vi "Process.vi"(8 "error in (no error)":errorcluster, 10 "Pound in":refnum<class "Pound.lvclass">, 11 "Qbus in":refnum<class "Qbus.lvclass">) -> (0 "error out":errorcluster)   [LabVIEW 2017, in "McsaAnalysisLowUpdate.lvlib"]
doc: "Calculates features, such as MCSA Speed and Rotor Bar Sideband, from waveforms that the channels in a data group acquire. Subsequent processes can evaluate this feature data to trigger alarms, collect data sets, and perform other operations."
uses:
  <vilib>/addons/InsightCM/Devices/Shared/Mcsa/McsaAnalysisLowUpdate/McsaAnalysisLowUpdate.lvlib
  <vilib>/addons/Qbus/Qbus.lvclass
  <vilib>/NI/Software Watchdog/Pound/Pound.lvclass
  <vilib>/addons/InsightCM/Devices/Shared/Mcsa/McsaAnalysisLowUpdate/controls/Config.ctl
  <vilib>/addons/InsightCM/Devices/Shared/Mcsa/McsaAnalysisLowUpdate/controls/Group.ctl
  <vilib>/addons/InsightCM/Utilities/Analysis/MCSA/controls/McsaLowUpdateChannel.ctl
  <vilib>/addons/InsightCM/Utilities/Analysis/Shared/controls/Feature.ctl
  <vilib>/addons/InsightCM/Utilities/Analysis/Shared/controls/AmplitudeScale.ctl
  <vilib>/addons/InsightCM/Utilities/Analysis/MCSA/controls/McsaMotor.ctl
  <vilib>/addons/InsightCM/Utilities/Analysis/MCSA/controls/McsaCalculationCache.ctl
  <vilib>/addons/Electrical Power/Motor Monitoring/subVIs/ep_Initial Conditions for MCSA Spectra.ctl
  <vilib>/addons/Electrical Power/Motor Monitoring/subVIs/ep_Demodulation Algorithm.ctl
  <vilib>/addons/Electrical Power/Motor Monitoring/subVIs/ep_Zoom FFT Settings.ctl
  <vilib>/addons/Electrical Power/Motor Monitoring/subVIs/ep_Initial Conditions for Speed Estimation.ctl
  <vilib>/NI/Software Watchdog/Watchdog/Watchdog.lvclass
  <vilib>/addons/InsightCM/Devices/Shared/Common/DataFlow/DataFlow.lvlib
  <vilib>/addons/InsightCM/Utilities/GlobalConfiguration/GlobalConfiguration.lvlib
  <vilib>/addons/InsightCM/Utilities/Analysis/Shared/AnalysisHelper.lvlib
  <vilib>/addons/InsightCM/Utilities/Analysis/MCSA/McsaAnalysisFunctions.lvlib
  <vilib>/addons/InsightCM/Devices/Shared/Mcsa/McsaResourceScheduler/McsaResourceScheduler.lvlib
  <vilib>/addons/Electrical Power/Motor Monitoring/NI_EP_Motor Monitoring.lvlib
  <vilib>/addons/TraceLogger/TraceLogger.lvlib
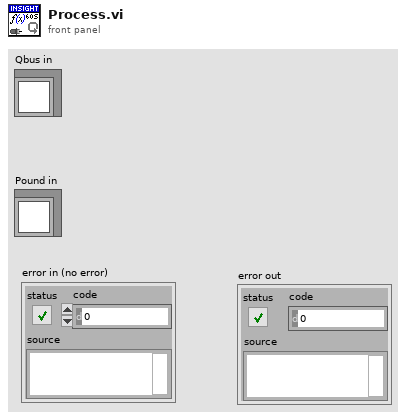
[diagram p1: front panel]
types:
  T1 = typedef "McsaAnalysisLowUpdate.lvlib/Config.ctl" = cluster{"Device Name":string, "Groups":T2[]}
  T2 = typedef "McsaAnalysisLowUpdate.lvlib/Group.ctl" = cluster{"Name":string, "Channels":T3[], "Motor Information":T6, "Calculation Cache":T7}
  T3 = typedef "McsaAnalysisFunctions.lvlib/McsaLowUpdateChannel.ctl" = cluster{"Name":string, "Id":string, "Type":string, "Wiring Configuration":string, "Nominal Voltage":dbl, "Phase A Channel":string, "Phase B Channel":string, "Phase C Channel":string, "Channel Status":string, "Features":T4[], "Data Valid":bool, "Acq Timestamp":timestamp}
  T4 = typedef "AnalysisHelper.lvlib/Feature.ctl" = cluster{"MetricType":string, "TdmsPropName":string, "DisplayName":string, "Unit":string, "Use Volts":bool, "Value":dbl, "Tag Id":string, "Properties":variant, "Amplitude Scale":T5, "valid":bool}
  T5 = typedef "AnalysisHelper.lvlib/AmplitudeScale.ctl" = enum16{"rms", "peak", "pk-pk"}
  T6 = typedef "McsaAnalysisFunctions.lvlib/McsaMotor.ctl" = cluster{"Model":string, "Manufacturer":string, "Serial Number":string, "Horsepower":dbl, "Horsepower Unit":string, "Full Load Speed":dbl, "Synchronous Speed":dbl, "Rated Volts":dbl, "Full Load Amps":dbl, "Frequency":dbl, "Service Factor":dbl, "Efficiency":dbl, "Efficiency @ 75% Load":dbl, "Efficiency @ 50% Load":dbl, "Efficiency @ 25% Load":dbl, "Power Factor":dbl, "VoltageBus":string, "VoltageBus ID":string, "Stator Resistance":dbl, "Estimate Stator Resistance":bool}
  T7 = typedef "McsaAnalysisFunctions.lvlib/McsaCalculationCache.ctl" = cluster{"Spectrum Reset":bool, "Spectrum":cluster{"f0":dbl, "df":dbl, "magnitude [dB]":dbl[]}, "max sideband magnitude [dB]":dbl, "rotor sideband step [Hz]":dbl, "spectrum initial conditions":T8, "Speed Reset":bool, "speed [RPM]":dbl, "slip":dbl, "speed initial conditions":T11, "line frequency [Hz]":dbl}
  T8 = typedef "NI_EP_Motor Monitoring.lvlib/ep_Initial Conditions for MCSA Spectra.ctl" = cluster{"hilbert state":cluster{"delay conditions":dbl[], "filter conditions":dbl[]}, "zoom FFT state":cluster{"phase state":dbl, "zoom FFT state":cluster{"zoom settings state":cluster{"zoom":i32, "stop band attenuation":enum16{"84 dB", "96 dB", "120 dB"}, "alias protect in final transition":bool, "oversampling ratio":dbl}, "SML Decimation Filter (complex input) state":cluster{"decimation settings state":cluster{"M":i32, "stop band attenuation":enum16{"84 dB", "96 dB", "120 dB"}, "alias protect in transition band":bool, "oversampling ratio":dbl}, "counter for garbage samples state":i32, "sml_Parameter Setting for Zoom Factor state":cluster{"filter length * interpolation state":i32, "interpolation state":i32, "comb filter order state":i32, "CFIR par state":cluster{"h":dbl[], "M":i32, "N":i32}, "LFIR par state":cluster{"h":dbl[], "M":i32, "N":i32}, "CIC Stages state":i32}, "aal_CIC (complex input) state":cluster{"aal_cascaded moving average (complex input) state":cluster{"states":cdb[], "circular buffers state":cdb[][], "circular buffer counter state":i32}, "aal_moving average with decimation by order (complex input) state":cluster{"residue result state":cdb, "processed data counter state":i32}}, "sml_Cascaded Decimation Filter (complex input) CFIR state":cluster{"unprocessed data state":cdb[], "final conditions state":cdb[][], "sml_M-1 Decimator with IC (complex input) state":cluster{"coefficients in reverse order state":dbl[], "max index for coefficients state":i32}}, "sml_Cascaded Decimation Filter (complex input) LFIR state":cluster{"unprocessed data state":cdb[], "final conditions state":cdb[][], "sml_M-1 Decimator with IC (complex input) state":cluster{"coefficients in reverse order state":dbl[], "max index for coefficients state":i32}}}, "ma_SML Data Packing (complex input) state":cluster{"array getting packed state":cdb[], "last array processed state":cdb[], "index state":i32, "packing parameters state":cluster{i32, "size":i32}}}, "FFT{X} [Vrms]":cdb[]}, "IIR filter state":cluster{"filter state":dbl[]}, "demodulation settings":cluster{"enable? (F)":bool, "algorithm":T9}, "highpass IIR Filter":cluster{"filter structure":enum32{"IIR 2nd Order", "IIR 4th Order"}, "Reverse Coefficients":dbl[], "Forward Coefficients":dbl[]}, "Hilbert FIR filter":cluster{"coefficients":dbl[], "delay":i32}, "zoom FFT settings":T10}
  T9 = typedef "NI_EP_Motor Monitoring.lvlib/ep_Demodulation Algorithm.ctl" = enum16{"1-phase signal", "3-phase signals"}
  T10 = typedef "NI_EP_Motor Monitoring.lvlib/ep_Zoom FFT Settings.ctl" = cluster{"FFT settings":cluster{"window":u16, "Window Size":i32, "FFT Size":i32, "%overlap":dbl}, "zoom settings":cluster{"zoom":i32, "stop band attenuation":enum16{"84 dB", "96 dB", "120 dB"}, "alias protect in final transition":bool, "oversampling ratio":dbl}, "other settings":cluster{"fmod":dbl, "f0":dbl, "df":dbl, "oidx":i32, "olen":i32}, "iterations":i32, "max block size":i32, "fs":dbl}
  T11 = typedef "NI_EP_Motor Monitoring.lvlib/ep_Initial Conditions for Speed Estimation.ctl" = cluster{"SVAF state":cluster{"space vector amplitude":dbl, "hilbert state":cluster{"delay conditions":dbl[], "filter conditions":dbl[]}}, "zoom FFT state":cluster{"phase state":dbl, "zoom FFT state":cluster{"zoom settings state":cluster{"zoom":i32, "stop band attenuation":enum16{"84 dB", "96 dB", "120 dB"}, "alias protect in final transition":bool, "oversampling ratio":dbl}, "SML Decimation Filter (complex input) state":cluster{"decimation settings state":cluster{"M":i32, "stop band attenuation":enum16{"84 dB", "96 dB", "120 dB"}, "alias protect in transition band":bool, "oversampling ratio":dbl}, "counter for garbage samples state":i32, "sml_Parameter Setting for Zoom Factor state":cluster{"filter length * interpolation state":i32, "interpolation state":i32, "comb filter order state":i32, "CFIR par state":cluster{"h":dbl[], "M":i32, "N":i32}, "LFIR par state":cluster{"h":dbl[], "M":i32, "N":i32}, "CIC Stages state":i32}, "aal_CIC (complex input) state":cluster{"aal_cascaded moving average (complex input) state":cluster{"states":cdb[], "circular buffers state":cdb[][], "circular buffer counter state":i32}, "aal_moving average with decimation by order (complex input) state":cluster{"residue result state":cdb, "processed data counter state":i32}}, "sml_Cascaded Decimation Filter (complex input) CFIR state":cluster{"unprocessed data state":cdb[], "final conditions state":cdb[][], "sml_M-1 Decimator with IC (complex input) state":cluster{"coefficients in reverse order state":dbl[], "max index for coefficients state":i32}}, "sml_Cascaded Decimation Filter (complex input) LFIR state":cluster{"unprocessed data state":cdb[], "final conditions state":cdb[][], "sml_M-1 Decimator with IC (complex input) state":cluster{"coefficients in reverse order state":dbl[], "max index for coefficients state":i32}}}, "ma_SML Data Packing (complex input) state":cluster{"array getting packed state":cdb[], "last array processed state":cdb[], "index state":i32, "packing parameters state":cluster{i32, "size":i32}}}, "FFT{X} [Vrms]":cdb[]}, "speed state":cluster{"speed [RPM]":dbl, "slip":dbl}, "speed estimation settings":cluster{"% overlap":dbl, "algorithm":T9}, "filter information":cluster{"coefficients":dbl[], "order":i32}, "zoom FFT settings":T10, "last valid window":i32, "fund. frequency for averager":dbl[]}
  T12 = typedef "DataFlow.lvlib/Data.ctl" = cluster{"DataGroup":string, "Waveforms":T13, "Map":T14, "Type":T15}
  T13 = typedef "wfmSGL_DVR.ctl" = refnum<data-value>
  T14 = typedef "PointValueMap.lvlib/PointMap.ctl" = refnum<data-value>
  T15 = typedef "DataFlow.lvlib/Type.ctl" = enum16{"High Rate", "Low Rate", "Burst Mode"}
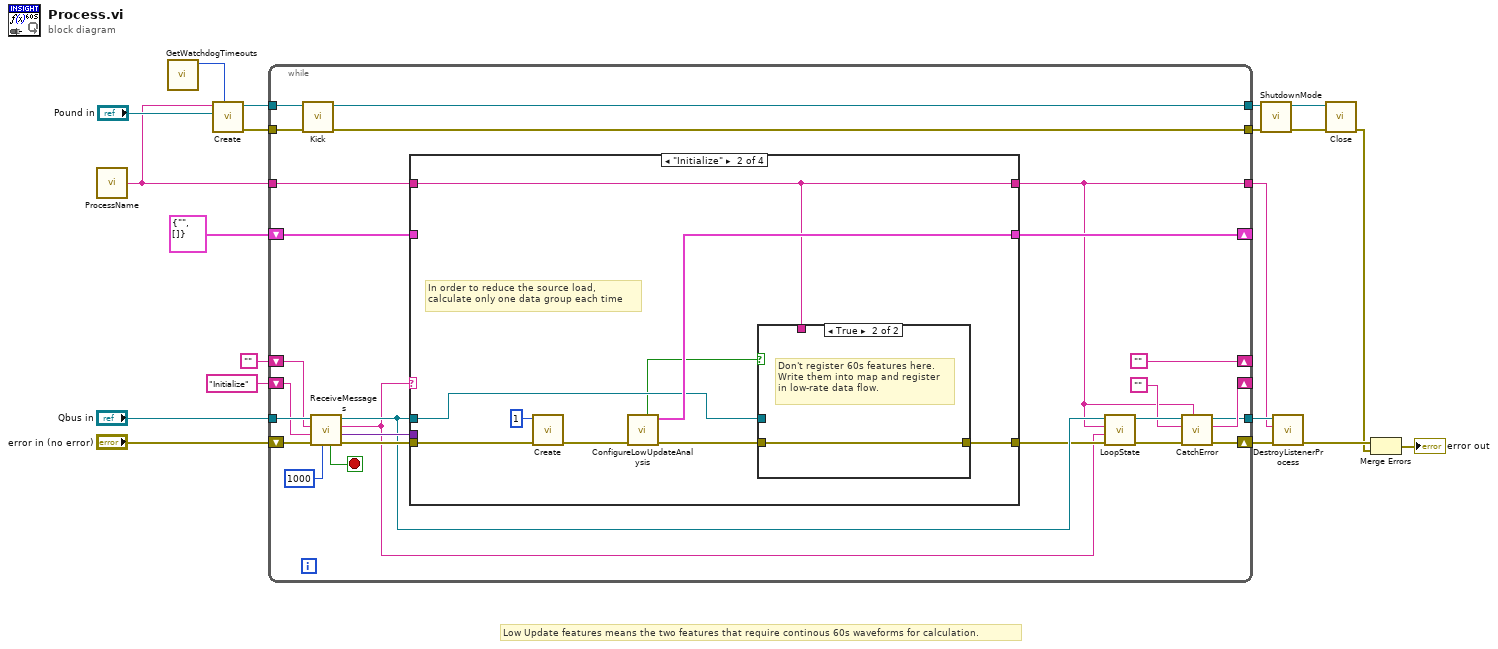
[diagram p0: block diagram]
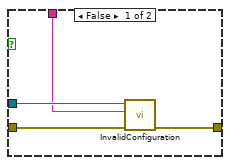
[diagram p3: hidden frame]
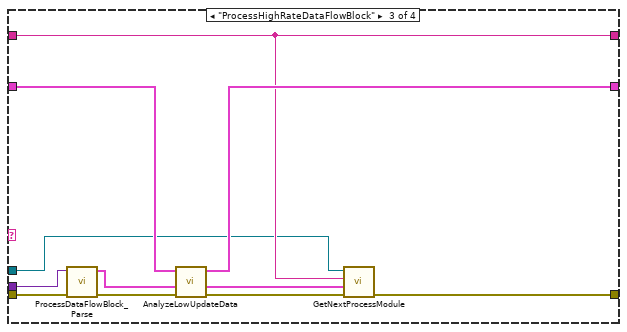
[diagram p4: hidden frame]
diagram:
  # "Low Update features means the two features that require continous 60s waveforms for calculation."
  n1 = call <vilib>:"ProcessName.vi"() -> ("ProcessName"=w2:string)  [unwired: 5 in]
  n2 = call <vilib>:"GetWatchdogTimeouts.vi"() -> ("software timeout"=w3:u32)  [unwired: 10 in, 1 out]
  n3 = call <vilib>:"Create.vi"("Execution Timeout (ms)"=w3, "Pound"="Pound in", "Name"=w2) -> ("error out"=w10:errorcluster, "Watchdog"=w11:refnum<data-value>)  [unwired: 7 in]
  n4 = while {
    shift-right: [""] -> _
    shift-left: "" -> [w40]
    shift-right: [w46] -> _
    shift-left: T1 {"Device Name"="", "Groups"=[]} ("Analysis Configuration") -> [w45]
    shift-right: [w27] -> _
    shift-left: "Initialize" ("MsgName") -> [w38]
    tunnel: w2 -> [w33]
    tunnel: [w26] -> w16
    tunnel: [w24] -> w15
    tunnel: "Qbus in" -> [w43]
    tunnel: [w37] -> w13
    tunnel: [w36] -> w12
    tunnel: w11 -> [w35]
    tunnel: w10 -> [w34]
    shift-right: [w25] -> w17
    shift-left: "error in (no error)" -> [w39]
    stop <- w22 stop-if-true
    n5 = call <vilib>:"Kick.vi"("error in (no error)"=w34, "Watchdog"=w35) -> ("error out"=w37:errorcluster, "Watchdog"=w36:refnum<data-value>)  [unwired: 8 in]
    n6 = call <vilib>:"ReceiveMessages.vi"("Timeout(100)"=1000, "error in (no error)"=w39, "Priority Action"=w38, "Default Action"=w40, "Qbus in"=w43) -> ("error out"=w41:errorcluster, "MsgValue"=w42:variant, "Action"=w23:string, "Qbus out"=w32:refnum<class "Qbus.lvclass">, "Exit"=w22:bool)  [unwired: 2 in]
    n7 = case shown="\"Initialize\"" w23 {
      tunnel: w41 -> [w49 w51 w72 w76]
      tunnel: [w49 w55 w67 w76] -> w31
      tunnel: w42 -> [_ _ w71 _]
      tunnel: [w48 w58 w73 w75] -> w46
      tunnel: w45 -> [w48 _ w74 w75]
      tunnel: w32 -> [_ w57 w66 _]
      tunnel: [w47 w53 w68 w77] -> w24
      tunnel: w33 -> [w47 w53 w68 w77]
      frame Default {
      }
      frame "Initialize" {
        # "In order to reduce the source load, \ncalculate only one data group each time"
        n8 = call <vilib>:"Create.vi"("error in (no error)"=w51, "count"=1) -> ("error out"=w50:errorcluster)  [unwired: 9 in]
        n9 = call <vilib>:"ConfigureLowUpdateAnalysis.vi"("error in (no error)"=w50) -> ("error out"=w56:errorcluster, "analysis config"=w58:T1, "all config found?"=w54:bool)  [unwired: 8 in]
        n10 = case shown="True" w54 {
          tunnel: w57 -> [w62 _]
          tunnel: w56 -> [w61 w63]
          tunnel: [w60 w63] -> w55
          tunnel: w53 -> [w59 _]
          frame False {
            n11 = call <vilib>:"InvalidConfiguration.vi"("error in (no error)"=w61, "description"=w59, "Qbus in"=w62) -> ("error out"=w60:errorcluster)  [unwired: 7 in, 1 out]
          }
          frame True {
            # "Don't register 60s features here.\nWrite them into map and register\nin low-rate data flow."
          }
        }
      }
      frame "ProcessHighRateDataFlowBlock" {
        n12 = call <vilib>:"ProcessDataFlowBlock_Parse.vi"("error in (no error)"=w72, "body"=w71) -> ("error out"=w65:errorcluster, "data"=w69:T12)  [unwired: 8 in]
        n13 = call <vilib>:"AnalyzeLowUpdateData.vi"("error in (no error)"=w65, "data in"=w69, "Analysis Configuration In"=w74) -> ("error out"=w64:errorcluster, "data out"=w70:T12, "Analysis Configuration Out"=w73:T1)  [unwired: 6 in]
        n14 = call <vilib>:"GetNextProcessModule.vi"("error in (no error)"=w64, "data"=w70, "source"=w68, "Qbus in"=w66) -> ("error out"=w67:errorcluster)  [unwired: 6 in, 1 out]
      }
      frame "Exit" {
      }
    }
    n15 = call <vilib>:"LoopState.vi"("error in (no error)"=w31, "loop action"=w23, "process name"=w24, "Qbus in"=w32) -> ("error out"=w28:errorcluster, "Qbus out"=w30:refnum<class "Qbus.lvclass">)  [unwired: 6 in]
    n16 = call <vilib>:"CatchError.vi"("source"=w24, "error in (no error)"=w28, "next action in"="", "Qbus in"=w30) -> ("error out"=w25:errorcluster, "next action out"=w27:string, "Qbus out"=w26:refnum<class "Qbus.lvclass">)  [unwired: 5 in]
  }
  n17 = call <vilib>:"ShutdownMode.vi"("error in (no error)"=w13, "Watchdog"=w12) -> ("error out"=w18:errorcluster, "Watchdog"=w19:refnum<data-value>)  [unwired: 8 in]
  n18 = call <vilib>:"DestroyListenerProcess.vi"("error in (no error)"=w17, "process name"=w15, "Qbus in"=w16) -> ("error in (no error)"=w9:errorcluster)  [unwired: 7 in, 1 out]
  n19 = call <vilib>:"Close.vi"("error in (no error)"=w18, "Watchdog"=w19) -> ("error out"=w8:errorcluster)  [unwired: 9 in]
  n20 = Merge Errors(w9, w8) -> (→"error out":errorcluster)
